vi "Requests.vi"(8 "error in (no error)":errorcluster, 9 "write enable":bool=TRUE, 11 "LIR-919 in":refnum<class "LIR-919D.lvclass">) -> (0 "error out":errorcluster, 3 "LIR-919 out":refnum<class "LIR-919D.lvclass">)   [LabVIEW 2021, in "LIR-919D.lvclass"]
uses:
  LIR-919D.lvclass
  D:/my_projects/projects/Algorithms/Labview/21/Modbus/MB_TCP2/MB_TCP.lvclass
  MB_TCP.lvclass/MB_TCP.ctl
  NI_modbus_upd/Ctl/Unit_ID.ctl
  NI_modbus_upd/TCP/TCP.lvclass/TCP.ctl
  NI_modbus_upd/Master Function Definition/Responses/Read Input Registers Response.vi
  NI_modbus_upd/Master network read write.vi
  NI_modbus_upd/Master Function Definition/Requests/Read Input Registers Request.vi
  NI_modbus_upd/Function data mismatch error1.vi
  NI_modbus_upd/Master Function Definition/Responses/Write Multiple Registers Response.vi
  NI_modbus_upd/Master Function Definition/Requests/Write Multiple Registers Request.vi
  NI_modbus_upd/Master Function Definition/Responses/Read Holding Registers Response.vi
  NI_modbus_upd/Master Function Definition/Requests/Read Holding Registers Request.vi
  NI_modbus_upd/Utility/Bytes to U16s1.vi
  NI_modbus_upd/Function code mismatch error1.vi
  NI_modbus_upd/Error Generator1.vi
  NI_modbus_upd/Read ADU Packet Master.vi
  NI_modbus_upd/Write ADU Packet Master.vi
  NI_modbus_upd/Modbus Data Unit (PDU)/Construct PDU1.vi
  NI_modbus_upd/Utility/U16s to Bytes1.vi
  NI_modbus_upd/Modbus Data Unit (PDU)/Unflatten to PDU1.vi
  NI_modbus_upd/TCP/Protocol Read.vi
  NI_modbus_upd/TCP/Protocol Write.vi
  <vilib>/Utility/error.llb/Clear Errors.vi
  NI_modbus_upd/Modbus Data Unit (PDU)/Deconstruct PDU1.vi
  NI_modbus_upd/TCP/TCP.lvclass
  ICPCON Registers/ICPCON Registers.lvlib
  MB_TCP.lvclass
  NI_modbus_upd/NI_modbus_upd.lvlib
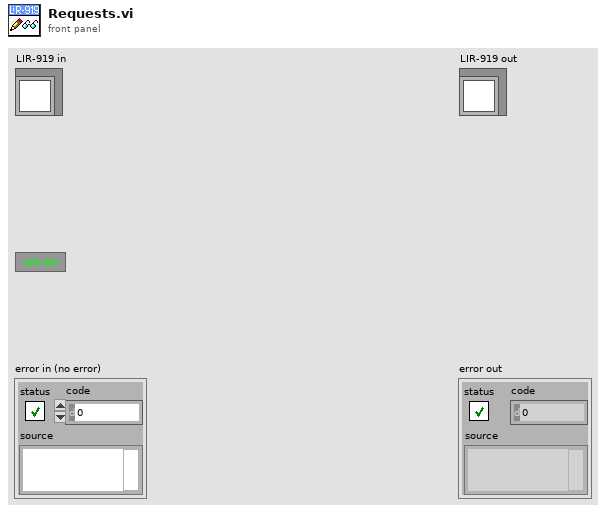
[diagram p1: front panel]
types:
  T1 = typedef "NI_modbus_upd.lvlib/Unit_ID.ctl" = cluster{"Protocol ID":u16, "Unit ID":u8}
  T2 = typedef "ICPCON Registers.lvlib/ICPCON Data.ctl" = cluster{"UTF":refnum<data-value>, "DI":refnum<data-value>, "DW":refnum<data-value>, "DO":refnum<data-value>, "IR":refnum<data-value>, "WR":refnum<data-value>, "OR":refnum<data-value>, "modified":refnum<data-value>}
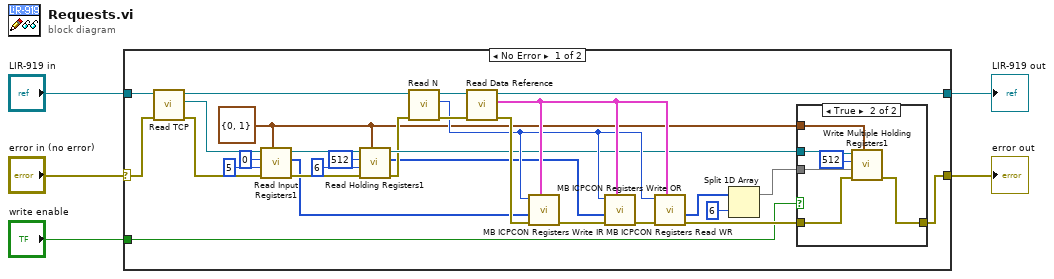
[diagram p0: block diagram]
diagram:
  n1 = case shown="No Error" "error in (no error)" {
    selector: "error in (no error)" -> [w27 w44]
    tunnel: [w24 w44] -> w3
    tunnel: [w26 w43] -> w4
    tunnel: "LIR-919 in" -> [w28 w43]
    tunnel: "write enable" -> [w6 _]
    frame No Error {
      w9 = T1 {"Protocol ID"=0, "Unit ID"=1} ("Unit_ID")
      n2 = call "Read TCP.vi"("error in (no error)"=w27, "MB_TCP in"=w28) -> ("error out"=w29:errorcluster, "TCP"=w31:refnum<class "TCP.lvclass">, "MB_TCP out"=w30:refnum<class "LIR-919D.lvclass">)  [unwired: 7 in]
      n3 = call "Read Input Registers1.vi"("Unit_ID"=w9, "error in (no error)"=w29, "number of input registers"=u16 5 ("number of discrete inputs"), "starting address"=u16 0, "Modbus master in"=w31) -> ("error out"=w13:errorcluster, "register values"=w7:u16[], "Modbus master out"=w15:refnum<class "TCP.lvclass">)  [unwired: 4 in]
      n4 = call "Read Holding Registers1.vi"("Unit_ID"=w9, "error in (no error)"=w13, "number of holding registers"=u16 6 ("number of discrete inputs"), "starting address"=u16 512, "Modbus master in"=w15) -> ("error out"=w12:errorcluster, "register values"=w8:u16[], "Modbus master out"=w14:refnum<class "TCP.lvclass">)  [unwired: 4 in]
      n5 = call "Read N.vi"("error in (no error)"=w12, "MB_TCP in"=w30) -> ("error out"=w34:errorcluster, "N"=w21:i32, "MB_TCP out"=w35:refnum<class "LIR-919D.lvclass">)  [unwired: 7 in]
      n6 = call "Read Data Reference.vi"("error in (no error)"=w34, "MB_TCP in"=w35) -> ("error out"=w22:errorcluster, "Data"=w25:T2, "MB_TCP out"=w26:refnum<class "LIR-919D.lvclass">)  [unwired: 7 in]
      n7 = call "MB ICPCON Registers Write IR.vi"("Data Reference"=w25, "error in (no error)"=w22, "Words In"=w7, "N"=w21) -> ("error out"=w23:errorcluster)  [unwired: 7 in]
      n8 = call "MB ICPCON Registers Write OR.vi"("Data Reference"=w25, "error in (no error)"=w23, "Words In"=w8, "N"=w21) -> ("error out"=w16:errorcluster)  [unwired: 7 in]
      n9 = call "MB ICPCON Registers Read WR.vi"("Data Reference"=w25, "error in (no error)"=w16, "N"=w21) -> ("error out"=w17:errorcluster, "Words out"=w19:u16[])  [unwired: 7 in]
      n10 = Split 1D Array(array=w19, index=6 ("length")) -> (first subarray=w18:u16[])  [unwired: 1 out]
      n11 = case shown="True" w6 {
        tunnel: w17 -> [w36 w41]
        tunnel: [w36 w39] -> w24
        tunnel: w14 -> [_ w42]
        tunnel: w9 -> [_ w38]
        tunnel: w18 -> [_ w37]
        frame False {
        }
        frame True {
          n12 = call "Write Multiple Holding Registers1.vi"("Unit_ID"=w38, "error in (no error)"=w41, "holding register values"=w37, "starting address"=u16 512, "Modbus master in"=w42) -> ("error out"=w39:errorcluster)  [unwired: 5 in, 1 out]
        }
      }
    }
    frame Error {
    }
  }
  "error out" <- w3
  "LIR-919 out" <- w4
